vi "Resize.vi"(8 "error in":errorcluster, 10 "length":dbl, 11 "Vec3d in":refnum<class "Vec3d.lvclass">) -> (0 "error out":errorcluster, 3 "Vec3d out":refnum<class "Vec3d.lvclass">)   [LabVIEW 2024, in "Vec3d.lvclass"]
uses:
  Vec3d.lvclass
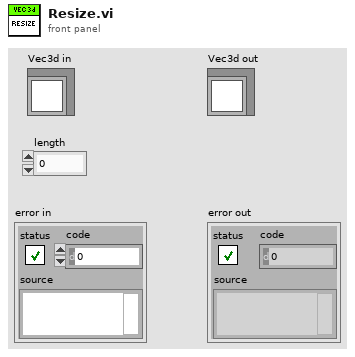
[diagram p1: front panel]
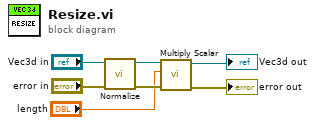
[diagram p0: block diagram]
diagram:
  n1 = call-dynamic "Normalize.vi"("error in"="error in", "Vec3d in"="Vec3d in") -> ("error out"=w6:errorcluster, "Vec3d out"=w5:refnum<class "Vec3d.lvclass">)  [unwired: 8 in]
  n2 = call-dynamic "Multiply Scalar.vi"("error in"=w6, "Scale"="length", "Vec3d in"=w5) -> ("error out"=→"error out":errorcluster, "Vec3d out"=→"Vec3d out":refnum<class "Vec3d.lvclass">)  [unwired: 7 in]
